vi "Colour Alternating Structures.vi"(6 "Variant in":variant, 7 "Shift Pressed?":bool, 8 "error in (no error)":errorcluster, 10 "QD Combo Box Ref":refnum<vi>, 11 "QD Launch VI Ref":refnum<vi>) -> (0 "error out":errorcluster, 4 "Variant out":variant)   [LabVIEW 2020]
doc: "Sets alternating diagram colours for nested structures to aid readability\n\nDefault Shortcut - [x]"
panel:
  in  "Undo Name":string="Quick Drop Keyboard Shortcut"
  # "Do not change the connector pane of this VI.\n\nSee the block diagram for directions on how to use this template."
  # "Specify the name of the Undo transaction"
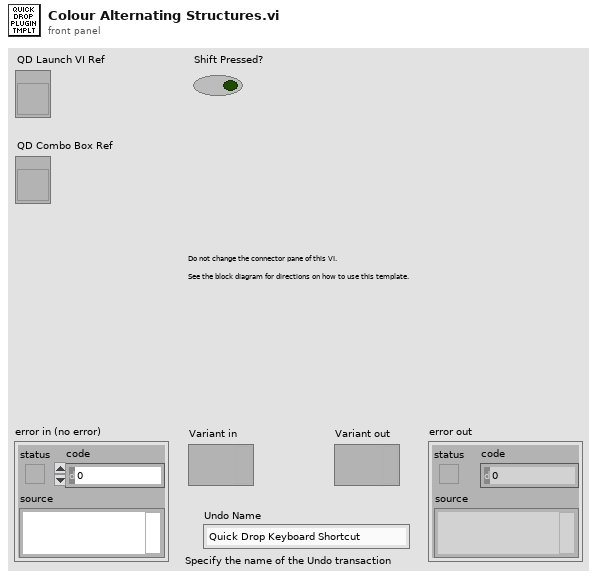
[diagram p1: front panel]
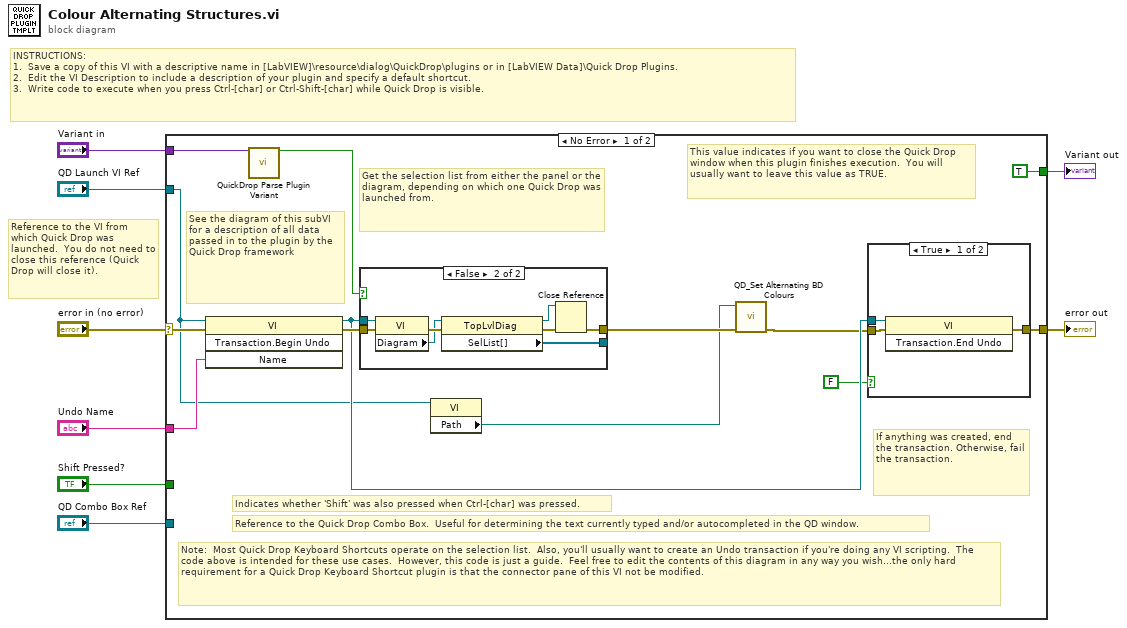
[diagram p0: block diagram]
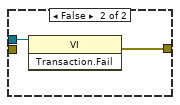
[diagram p2: hidden frame]
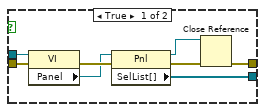
[diagram p3: hidden frame]
diagram:
  # "Reference to the VI from which Quick Drop was launched.  You do not need to close this reference (Quick Drop will close it)."
  # "INSTRUCTIONS:\n1.  Save a copy of this VI with a descriptive name in [LabVIEW]\\resource\\dialog\\QuickDrop\\plugins or in [LabVIEW Data]\\Quick Drop Plugins.\n2.  Edit the VI Description to include a description of your plugin and specify a default shortcut. \n3.  Write code to execute when you press Ctrl-[char] or Ctrl-Shift-[char] while Quick Drop is visible."
  n1 = case shown="No Error" "error in (no error)" {
    selector: "error in (no error)" -> [w20 w43]
    tunnel: [w15 w43] -> w7
    tunnel: "QD Launch VI Ref" -> [w10 _]
    tunnel: "Shift Pressed?" -> [_ _]
    tunnel: "QD Combo Box Ref" -> [_ _]
    tunnel: "Variant in" -> [w21 _]
    tunnel: "Undo Name" -> [w19 _]
    tunnel: [TRUE _] -> w1
    frame No Error {
      # "Note:  Most Quick Drop Keyboard Shortcuts operate on the selection list.  Also, you'll usually want to create an Undo transaction if you're doing any VI scripting.  The code above is intended for these use cases.  However, this code is just a guide.  Feel free to edit the contents of this diagram in any way you wish...the only hard requirement for a Quick Drop Keyboard Shortcut plugin is that the connector pane of this VI not be modified."
      # "Get the selection list from either the panel or the diagram, depending on which one Quick Drop was launched from."
      # "If anything was created, end the transaction. Otherwise, fail the transaction."
      # "This value indicates if you want to close the Quick Drop window when this plugin finishes execution.  You will usually want to leave this value as TRUE."
      # "See the diagram of this subVI for a description of all data passed in to the plugin by the Quick Drop framework"
      # "Reference to the Quick Drop Combo Box.  Useful for determining the text currently typed and/or autocompleted in the QD window."
      # "Indicates whether 'Shift' was also pressed when Ctrl-[char] was pressed."
      n2 = invoke class="VI" method="Transaction.Begin Undo"(reference=w10, error in=w20, "Name"=w19) -> (reference out=w14:refnum<vi>, error out=w16:errorcluster)  [unwired: 1 in, 2 out]
      n3 = call <vilib>:"QuickDrop Parse Plugin Variant.vi"("QDKS Variant in"=w21) -> ("QD Launch VI Panel?"=w17:bool)  [unwired: 12 in, 2 out]
      n4 = case shown="False" w17 {
        tunnel: w16 -> [w34 w42]
        tunnel: w14 -> [w33 w41]
        tunnel: [w28 w36] -> w12
        tunnel: [w27 w35] -> _
        frame True {
          n5 = property class="VI"(reference=w33, error in=w34) -> (error out=w32:errorcluster, "Panel"=w31:refnum<vi>)  [unwired: 1 out]
          n6 = property class="Pnl"(reference=w31, error in=w32) -> (reference out=w29:refnum<vi>, error out=w30:errorcluster, "SelList[]"=w27:refnum<vi>[])
          n7 = Close Reference(reference=w29, error in (no error)=w30) -> (error out=w28:errorcluster)
        }
        frame False {
          n8 = property class="VI"(reference=w41, error in=w42) -> (error out=w40:errorcluster, "Diagram"=w39:refnum<vi>)  [unwired: 1 out]
          n9 = property class="TopLvlDiag"(reference=w39, error in=w40) -> (reference out=w37:refnum<vi>, error out=w38:errorcluster, "SelList[]"=w35:refnum<vi>[])
          n10 = Close Reference(reference=w37, error in (no error)=w38) -> (error out=w36:errorcluster)
        }
      }
      n11 = property class="VI"(reference=w10) -> ("Path"=w9:path)  [unwired: 1 in, 2 out]
      n12 = call <resource>:"QD_Set Alternating BD Colours.vi"("error in (no error)"=w12, "Path"=w9) -> ("error out"=w11:errorcluster)  [unwired: 9 in]
      n13 = case shown="True" FALSE {
        tunnel: w14 -> [w23 w25]
        tunnel: [w24 w26] -> w15
        tunnel: w11 -> [w22 _]
        frame True {
          n14 = invoke class="VI" method="Transaction.End Undo"(reference=w23, error in=w22) -> (error out=w24:errorcluster)  [unwired: 1 in, 2 out]
        }
        frame False {
          n15 = invoke class="VI" method="Transaction.Fail"(reference=w25) -> (error out=w26:errorcluster)  [unwired: 2 in, 2 out]
        }
      }
    }
    frame Error {
    }
  }
  "error out" <- w7
  "Variant out" <- w1
